vi "niRFSysCalReader Cal Data Variant Name.vi"(9 "Power (dBm)":dbl, 11 "Frequency (Hz)":dbl) -> (3 "Calibration Data Name":string)   [LabVIEW 2016, in "niRFSysCalReader.lvlib"]
doc: "Returns the variant attribute name for the cal data"
uses:
  niRFSysCalReader.lvlib
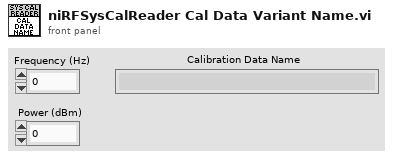
[diagram p1: front panel]
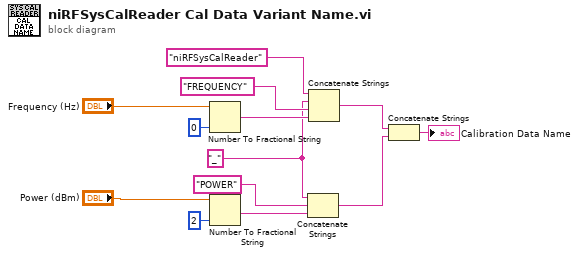
[diagram p0: block diagram]
diagram:
  w1 = "_" ("string")
  n1 = Number To Fractional String(number="Frequency (Hz)", precision (6)=i16 0) -> (F-format string=w9:string)  [unwired: 2 in]
  n2 = Number To Fractional String(number="Power (dBm)", precision (6)=i16 2) -> (F-format string=w6:string)  [unwired: 2 in]
  n3 = Concatenate Strings(w1, "POWER" ("string"), w6) -> (w4:string)
  n4 = Concatenate Strings("niRFSysCalReader" ("string"), w1, "FREQUENCY" ("string"), w9) -> (w5:string)
  n5 = Concatenate Strings(w5, w4) -> (→"Calibration Data Name":string)
